vi "Robot Global Data.vi"() -> ()   [LabVIEW 2012]
doc: "This global VI can contain as many global variables as you need. Place a control on the panel, give it a good name. To read or write to it from a VI, drag the icon to the diagram of that VI. You can also drag from the project. Click on the node to change which global you access. You shouldn't have multiple locations writing to a global or it will cause a race-condition."
uses:
  <vilib>/Rock Robotics/WPI/Camera/WPI_CameraImageSize.ctl
  <vilib>/Rock Robotics/WPI/DriverStation/WPI_DriverStationRobotMode2.ctl
panel:
  in  "oldScrewValue":dbl
  in  "zPos":dbl=16.5
  in  "oldValue":i32
  in  "ballScrewAutoFlag":i8
  in  "shootAutoFlag":i8
  in  "numBalls":i8
  in  "topFlag":i8
  in  "botFlag":i8
  in  "c":i8
  in  "readyToShoot":u8
  in  "shootMode":u8
  in  "ShooterSpeed":dbl=1000.0
  in  "ShooterKillCounter":dbl
  in  "buttonPrevValue":i8
  in  "ShooterOnOff":i8=1
  in  "timerCounter":dbl
  in  "ballScrewPosition":dbl=0.55
  in  "killBallScrewFlag":i8
  in  "killDriveTrainFlag":i8
  in  "beltCase":i8=3
  in  "shootFlag":u8=1
  in  "ShooterKillFlag":u8
  out "Target Info":T1(array[cluster])
  in  "Robot Mode":T2
  in  "LED toggle rate (ms)":u32=20
  in  "image size":T3=enum."320x240"
  in  "Enable Vision":bool=TRUE
  # "USED IN BELT CONTROL"
  # "USED IN SHOOTER CONTROL"
  # "USED IN DRIVETRAIN CONTROL"
  # "USED IN BALL SCREW CONTROL"
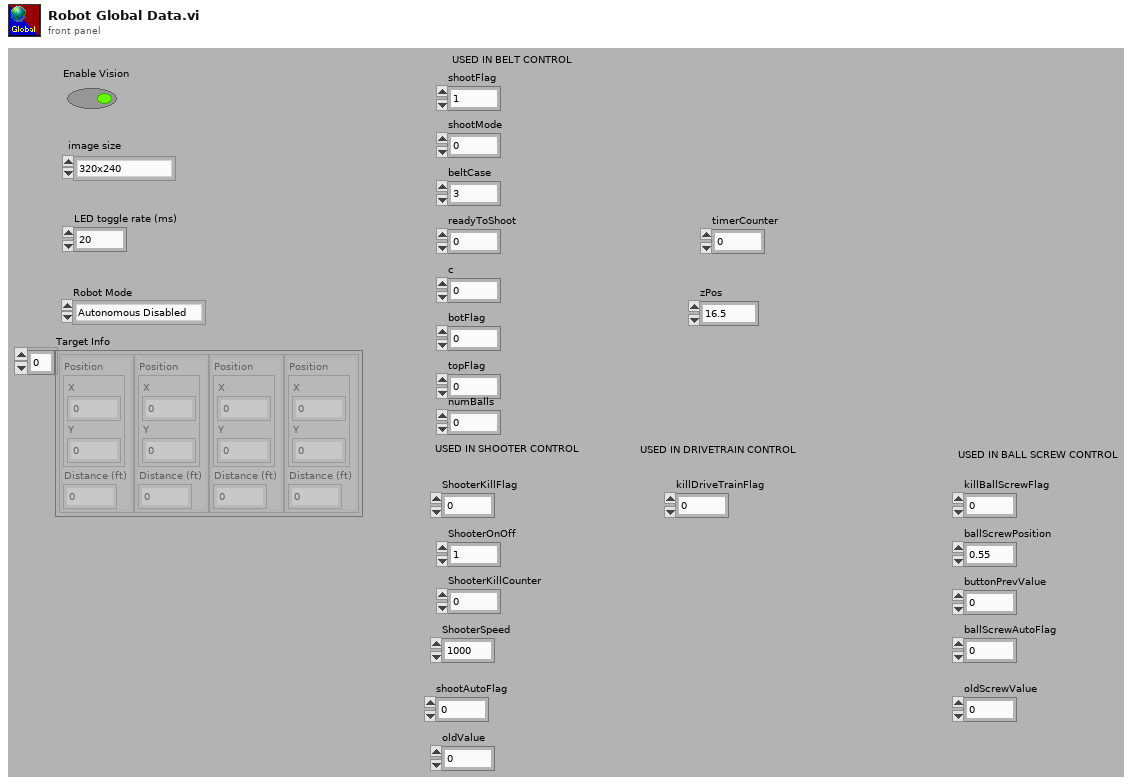
[diagram p1: front panel]
types:
  T1 = cluster{"Position":cluster{"X":dbl, "Y":dbl}, "Distance (ft)":dbl}[]
  T2 = typedef "WPI_DriverStationRobotMode2.ctl" = enum16{"Autonomous Disabled", "Autonomous Enabled", "Teleop Disabled", "Teleop Enabled", "Timeout", "Finish", "Test Disabled", "Test Enabled"}
  T3 = typedef "WPI_CameraImageSize.ctl" = enum16{"640x480", "320x240", "160x120"}
diagram:
